vi "TIScaleOverlay.vi"(6 "plotInfoArray":T1(array[cluster]), 7 "\"At\" location":T2={"XcoordSys"="graph", "YcoordSys"="graph", "Xvalue"=0.05, "Yvalue"=0.92}, 9 "Scale":dbl=300.0 caption="Scale 1:" min=1.0 max=10000.0 step=50.0) -> (3 "gnuplotOut":string)   [LabVIEW 2013]
uses:
  at.ctl
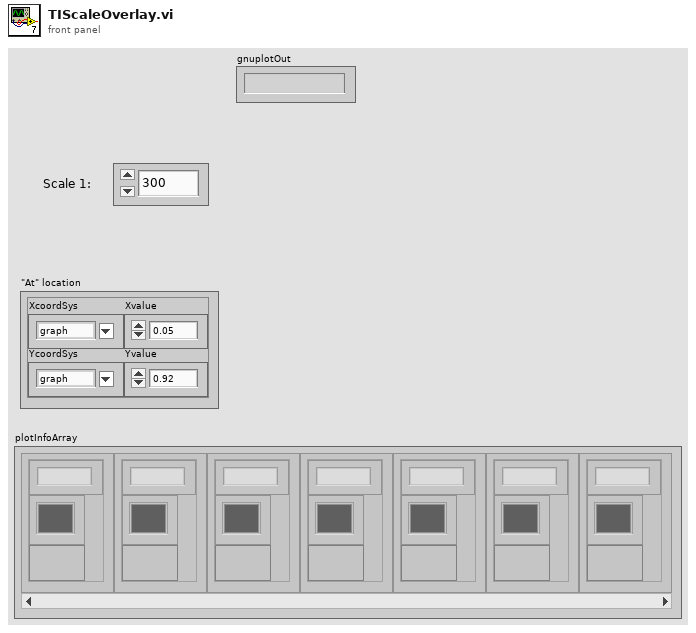
[diagram p1: front panel]
types:
  T1 = cluster{"Plot Name":string, "Plot.Plot Color":u32, "Plot.Visible?":bool}[]
  T2 = typedef "at.ctl" = cluster{"XcoordSys":string, "YcoordSys":string, "Xvalue":dbl, "Yvalue":dbl}
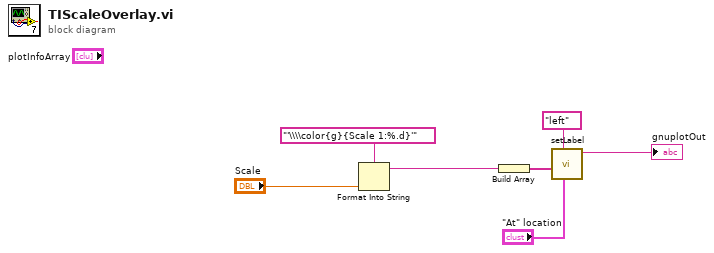
[diagram p0: block diagram]
diagram:
  n1 = Format Into String(format string="'\\\\color{g}{Scale 1:%.d}'", "Scale") -> (resulting string=w3:string)  [unwired: 2 in, 1 out]
  n2 = Build Array(w3) -> (w4:string[])
  n3 = call "setLabel.vi"("\"At\" location"="\"At\" location", "Justify"="left", "multilineLabel"=w4) -> ("String out"=→"gnuplotOut":string)  [unwired: 7 in, 1 out]
